vi "Inverse Fast Hilbert Transform.vi"(0 "X":dbl[](array[numeric])) -> (1 "Inv Hilbert {X}":dbl[](array[numeric]), 2 "error":i32)   [LabVIEW 2017, in "NI_AALPro.lvlib"]
doc: "Computes the inverse fast Hilbert transform of the input sequence <B>X</B> using Fourier identities."
uses:
  <vilib>/Analysis/NI_AALPro.lvlib
  <resource>/lvanlys.dll
panel:
  # "Inverse Fast Hilbert Transform"
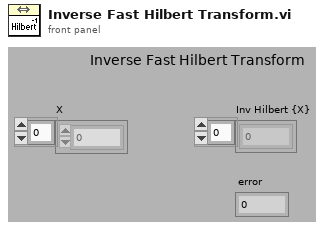
[diagram p1: front panel]
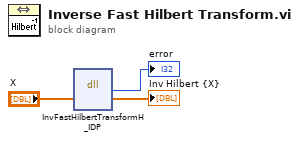
[diagram p0: block diagram]
diagram:
  n1 = dll-call lib="e:/builds/penguin/labview/branches/2017/dev/dist/resource/lvanlys.*" fn="InvFastHilbertTransformH_IDP"("xH"="X") -> ("return type"=→"error":i32, "xH"=→"Inv Hilbert {X}":dbl[])  [unwired: 5 in, 2 out]
